vi "Move Into Block Diagram Object.vi"() -> ()   [LabVIEW 2023]
doc: "Demonstrates the Move method in VI Scripting to programmatically move an object from one location to another, where the destination is a structure on the block diagram."
uses:
  <vilib>/Utility/miscctls.llb/LVPositionTypeDef.ctl
panel:
  in  "For Loop Label":string="Destination For Loop"
  in  "Add Label":string="Move Me - Add"
  # "Overview: Demonstrates the Move method in VI Scripting to programmatically move an object from one location to another.\nInstructions:\n1. Open the block diagrams of Test - Moving Objects Source.vi and Test - Moving Objects Target.vi.\n2. Run this VI. The \"Move Me - Add\" function will be copied from the source VI into the For Loop in the target VI.\n\nNote: When moving an object from one VI to another, the operation results in a copy, since the original object is preserved. When moving an object to a different location in the same VI, it will not be a copy operation unless the Duplicate? parameter of the Move method is set to TRUE."
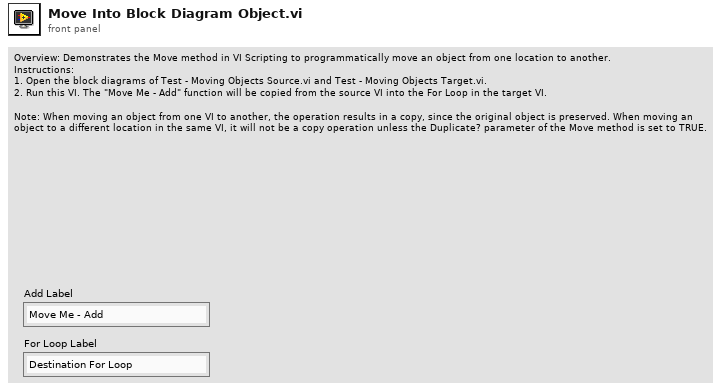
[diagram p1: front panel]
types:
  T1 = typedef "LVPositionTypeDef.ctl" = cluster{"Left":i32, "Top":i32}
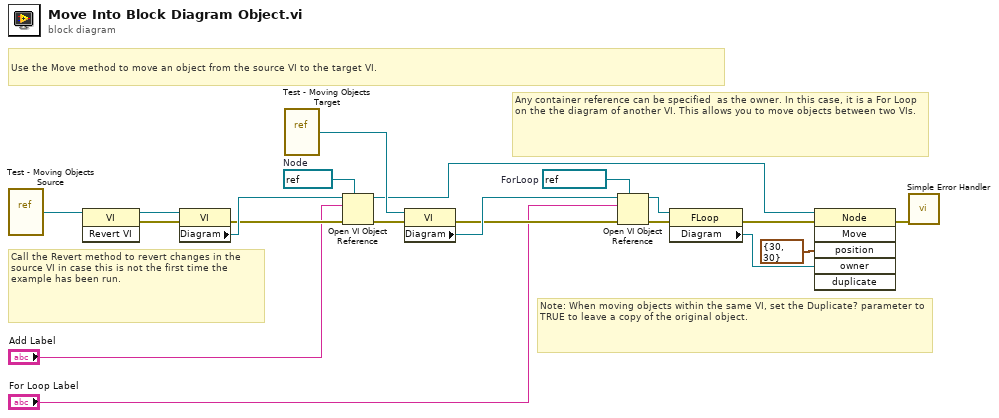
[diagram p0: block diagram]
diagram:
  w5 = refnum<vi> refnum  # ForLoop
  w7 = refnum<vi> refnum  # Node
  # "Note: When moving objects within the same VI, set the Duplicate? parameter to TRUE to leave a copy of the original object."
  # "Any container reference can be specified  as the owner. In this case, it is a For Loop on the the diagram of another VI. This allows you to move objects between two VIs."
  # "Call the Revert method to revert changes in the source VI in case this is not the first time the example has been run."
  # "Use the Move method to move an object from the source VI to the target VI."
  n1 = vi-ref "Test - Moving Objects Source.vi"() -> (w20:refnum<vi>)
  n2 = invoke class="VI" method="Revert VI"(reference=w20) -> (reference out=w18:refnum<vi>, error out=w17:errorcluster)  [unwired: 2 in, 1 out]
  n3 = property class="VI"(reference=w18, error in=w17) -> (error out=w11:errorcluster, "Diagram"=w15:refnum<vi>)  [unwired: 1 out]
  n4 = vi-ref "Test - Moving Objects Target.vi"() -> (w19:refnum<vi>)
  n5 = Open VI Object Reference(7:w7, 8:w11, 10:"Add Label", 11:w15) -> (0:w10:errorcluster, 3:w1:refnum<vi>)
  n6 = property class="VI"(reference=w19, error in=w10) -> (error out=w9:errorcluster, "Diagram"=w13:refnum<vi>)  [unwired: 1 out]
  n7 = Open VI Object Reference(7:w5, 8:w9, 10:"For Loop Label", 11:w13) -> (0:w2:errorcluster, 3:w3:refnum<vi>)
  n8 = property class="FLoop"(reference=w3, error in=w2) -> (error out=w8:errorcluster, "Diagram"=w12:refnum<vi>)  [unwired: 1 out]
  n9 = invoke class="Node" method="Move"(reference=w1, error in=w8, "position"=T1 {"Left"=30, "Top"=30}, "owner"=w12) -> (error out=w16:errorcluster)  [unwired: 2 in, 5 out]
  n10 = call <vilib>:"Simple Error Handler.vi"("error in (no error)"=w16) -> ()  [unwired: 4 in, 5 out]
